vi "Save VI.vi"(8 "error in":errorcluster, 11 "vi ref in":refnum<vi>) -> (0 "error out":errorcluster, 3 "vi ref out":refnum<vi>)   [LabVIEW 2020, in "Build Automation.lvlib"]
uses:
  Build Automation.lvlib
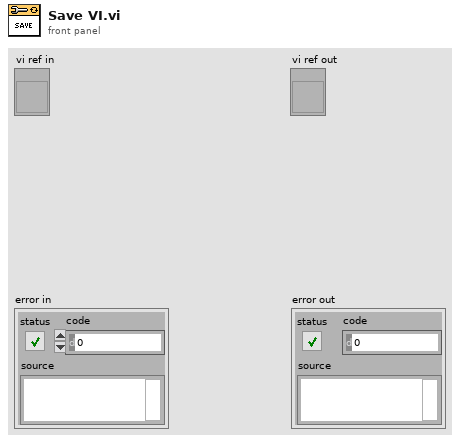
[diagram p1: front panel]
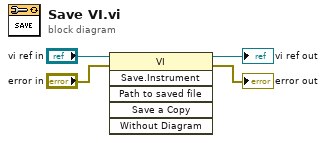
[diagram p0: block diagram]
diagram:
  n1 = invoke class="VI" method="Save.Instrument"(reference="vi ref in", error in="error in") -> (reference out=→"vi ref out":refnum<vi>, error out=→"error out":errorcluster)  [unwired: 4 in, 4 out]
